vi "painting_controller_a.vi"(0 "In Bounds":bool, 1 "Mouse Clicked":bool, 2 "Old Point":cluster{"X":i32, "Y":i32}, 3 "New Point":cluster{"X":i32, "Y":i32}, 4 "Was Painting":bool) -> (5 "Split":bool, 6 "Painting":bool, 7 "Add Point":bool)   [LabVIEW 2017]
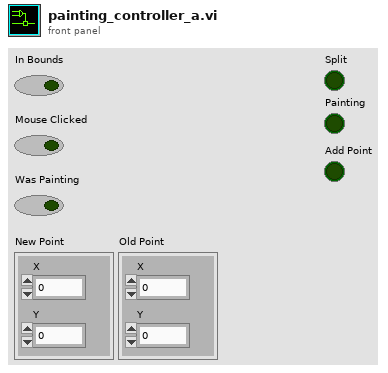
[diagram p1: front panel]
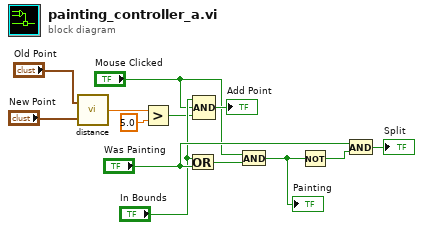
[diagram p0: block diagram]
diagram:
  n1 = call "distance.vi"("Point B"="New Point", "Point A"="Old Point") -> ("Distance"=w4:dbl)
  n2 = Greater?(x=w4, y=5.0) -> (0:w3:bool)
  n3 = Or(x="In Bounds", y="Was Painting") -> (x .or. y?=w10:bool)
  n4 = Compound Arithmetic op=AND("In Bounds", "Mouse Clicked", w3) -> (→"Add Point":bool)
  n5 = And(x="Mouse Clicked", y=w10) -> (x .and. y?=w11:bool)
  "Painting" <- w11
  n6 = Not(x=w11) -> (.not. x?=w12:bool)
  n7 = And(x="Was Painting", y=w12) -> (x .and. y?=→"Split":bool)
